vi "HE_state.vi"(6 "ZB":bool[](array[boolean])=[FALSE, FALSE], 7 "Alarm":bool[](array[boolean])=[FALSE, FALSE], 9 "XB":bool[](array[boolean])=[FALSE, FALSE, FALSE, FALSE, FALSE], 10 "Z_control":T5={"Z_HSw"=1, "Z_HSetState"=enum."on", "Z_ASetState"=enum."on", "Z_DSetState"=enum."on"}, 11 "HE_state_in":refnum<class "HE_state_v2.lvclass">) -> (1 "YB":bool[](array[boolean]), 2 "Z":T1={"Z_Source"=enum."local disabled", "Z_SetState"=enum."on", "Z_State"=enum."alarm", "Z_State_T"=0, "ZM_State"=enum."initialization", "ZM_State_T"=0, "ALR  L1"=FALSE, "ALR  L2"=FALSE, "HH_run"=0}, 3 "HE_state_out":refnum<class "HE_state_v2.lvclass">, 5 "ALR_ON":bool[](array[boolean]))   [LabVIEW 2019, in "Heating.lvlib" / "HE_state_v2.lvclass"]
uses:
  HE_state_v2.lvclass
  Heating.lvlib
  ctl/ZM_State.ctl
  ctl/Z_State.ctl
  ctl/Z_source.ctl
  ctl/Z.ctl
  ZM_state/HE_ZM_state.lvclass
  Z_state_v2/HE_Z_state_v2.lvclass
  C:/my_projects/projects/Algorithms/Labview/19/Heating/heating1/Z_state_v2/HE_Z_state_v2.lvclass
  C:/my_projects/projects/Algorithms/Labview/19/Heating/heating1/ZM_state/HE_ZM_state.lvclass
  C:/my_projects/projects/Algorithms/Labview/19/Sequence/State/State.lvclass
  ctl/Z_control.ctl
panel:
  # "Alarm_L1"
  # "Alarm_L2"
  # "Ki_XB01 contactor on"
  # "Ki_XB02 contactor off"
  # "XB24 local hand on"
  # "heating end"
  # "cooling end"
  # "Ki_ZB01 contactor on reg"
  # "Ki_ZB02 contactor off reg"
  # "TsStop"
  # "T_check"
  # "T_start_delay"
  # "T_heat_start"
  # "T_stop_delay"
  # "T_set_min"
  # "T_heat_stop"
  # "T_restart_delay"
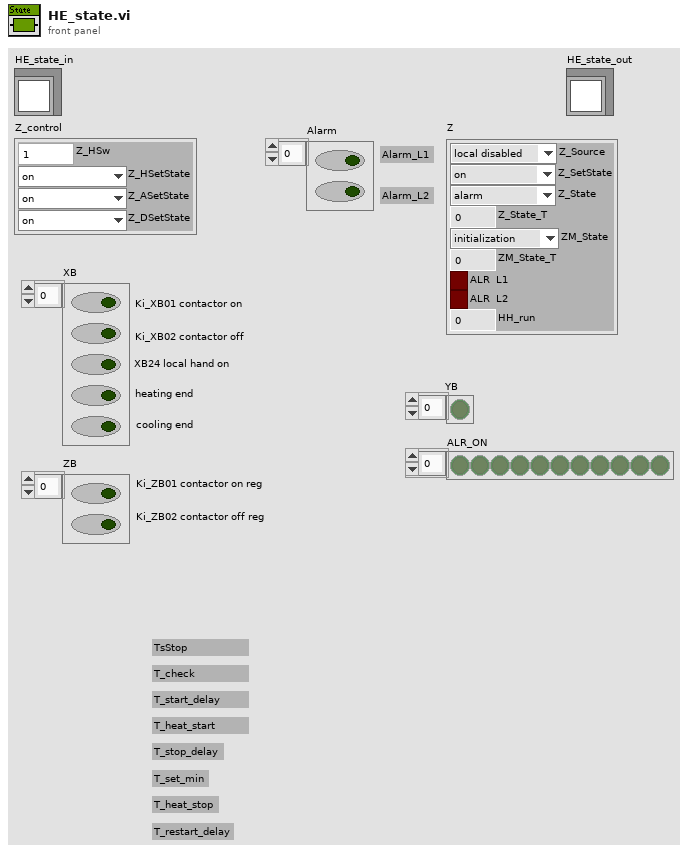
[diagram p1: front panel]
types:
  T1 = typedef "Heating.lvlib/Z.ctl" = cluster{"Z_Source":T2, "Z_SetState":T3, "Z_State":T3, "Z_State_T":u32, "ZM_State":T4, "ZM_State_T":u32, "ALR  L1":bool, "ALR  L2":bool, "HH_run":u64}
  T2 = typedef "Heating.lvlib/Z_source.ctl" = enum8{"initialize", "local disabled", "local hand", "hand", "auto", "dist"}
  T3 = typedef "Heating.lvlib/Z_State.ctl" = enum8{"initialization", "alarm", "disabled", "not ready", "stop ready", "reserv", "switched off", "reserv2", "switched on", "check", "on min", "decrease out", "on", "increase out", "on max"}
  T4 = typedef "Heating.lvlib/ZM_State.ctl" = enum8{"initialization", "stop", "start_cmd", "contactor_on_cmd", "heating", "on", "stop_cmd", "power_down", "contactor_off_cmd", "cooling", "restart_delay"}
  T5 = typedef "Heating.lvlib/Z_control.ctl" = cluster{"Z_HSw":u8, "Z_HSetState":T3, "Z_ASetState":T3, "Z_DSetState":T3}
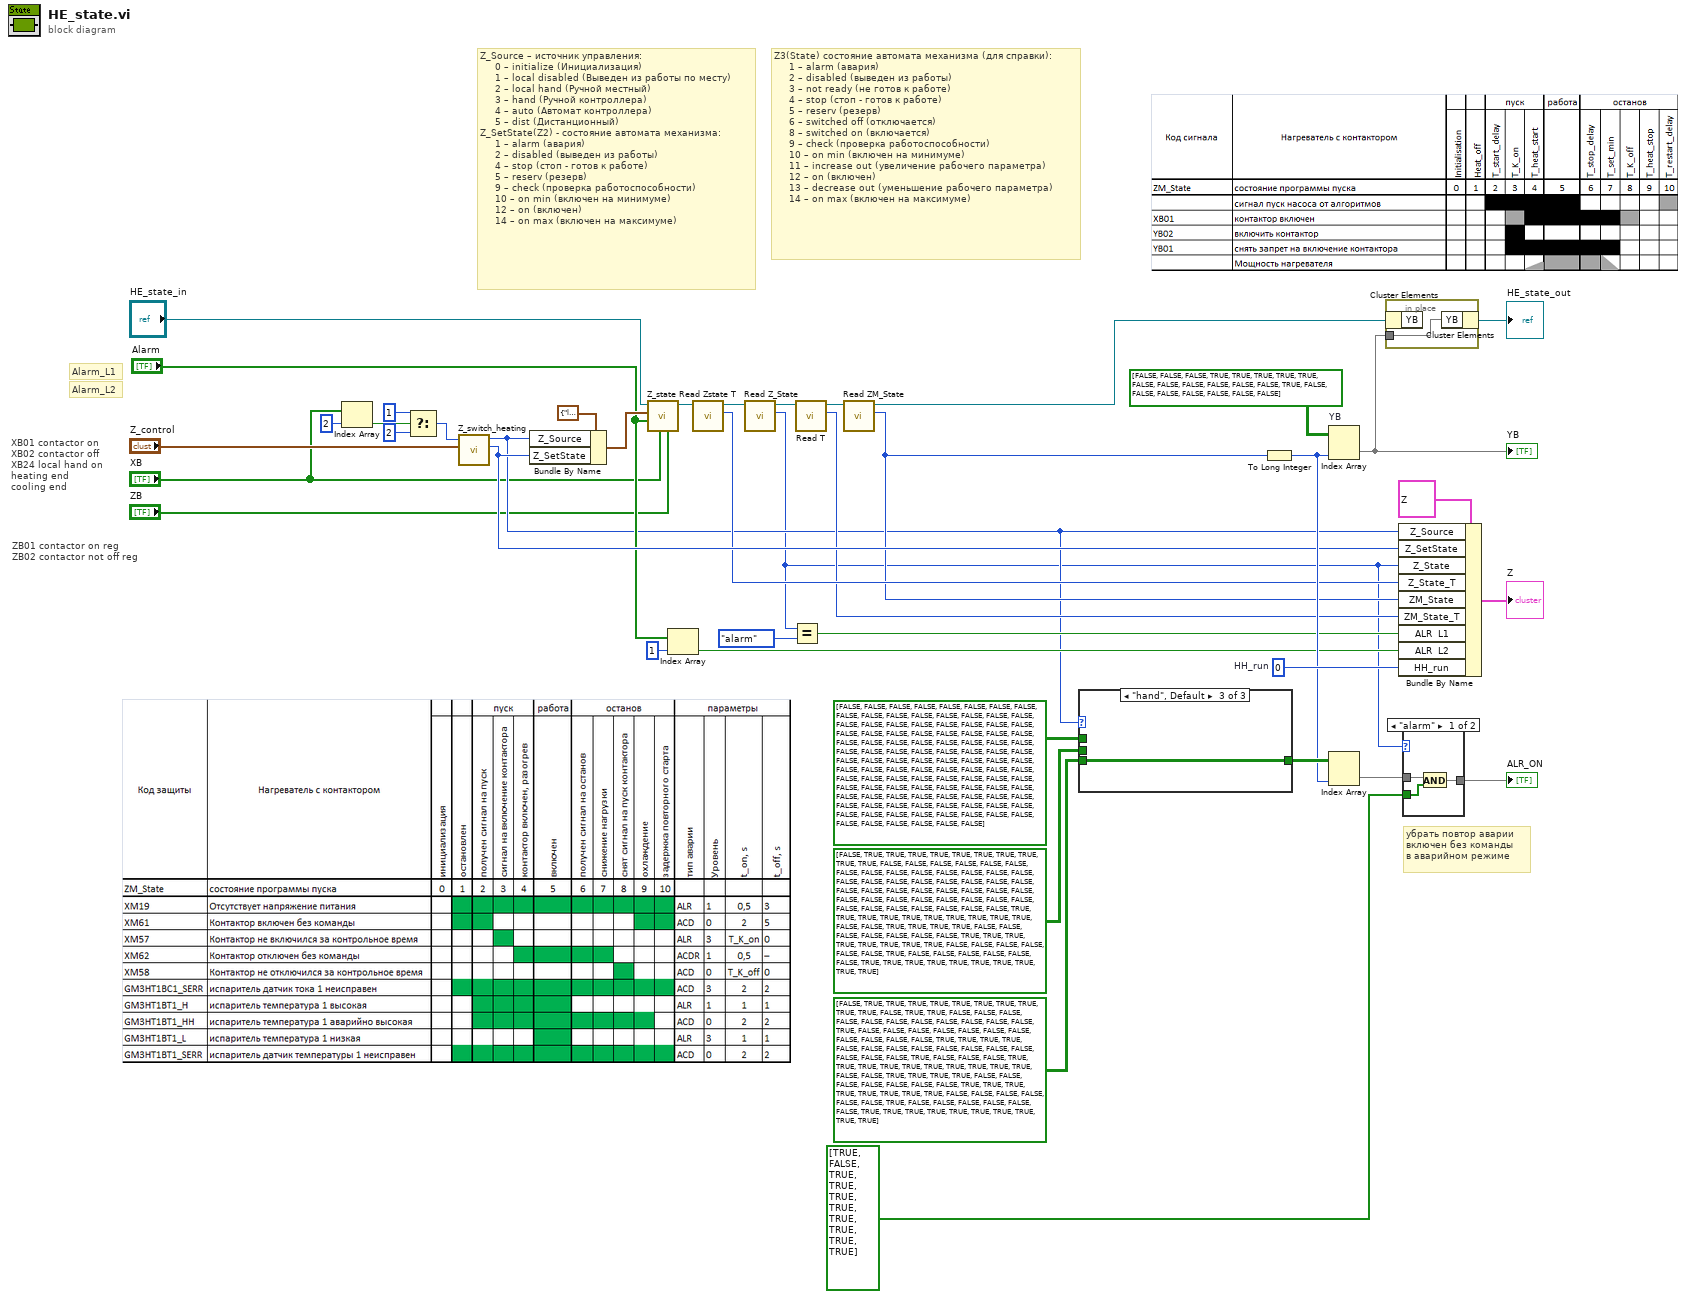
[diagram p0: block diagram]
diagram:
  w25 = 0  # HH_run
  # "Alarm_L2"
  # "Alarm_L1"
  # "ZB01 contactor on reg\nZB02 contactor not off reg"
  # "XB01 contactor on\nXB02 contactor off\nXB24 local hand on\nheating end\ncooling end"
  # "убрать повтор аварии\nвключен без команды\nв аварийном режиме"
  # "Z_Source – источник управления:\n     0 – initialize (Инициализация)\n     1 – local disabled (Выведен из работы по месту)\n     2 – local hand (Ручной местный)\n     3 – hand (Ручной контроллера)\n     4 – auto (Автомат контроллера)\n     5 – dist (Дистанционный)\nZ_SetState(Z2) - состояние автомата механизма:\n     1 – alarm (авария)\n     2 – disabled (выведен из работы)\n     4 – stop (стоп - готов к работе)\n     5 – reserv (резерв)\n     9 – check (проверка работоспособности)\n     10 – on min (включен на минимуме)\n     12 – on (включен)\n     14 – on max (включен на максимуме)"
  # "Z3(State) состояние автомата механизма (для справки):\n     1 – alarm (авария)\n     2 – disabled (выведен из работы)\n     3 – not ready (не готов к работе)\n     4 – stop (стоп - готов к работе)\n     5 – reserv (резерв)\n     6 – switched off (отключается)\n     8 – switched on (включается)\n     9 – check (проверка работоспособности)\n     10 – on min (включен на минимуме)\n     11 – increase out (увеличение рабочего параметра)\n     12 – on (включен)\n     13 – decrease out (уменьшение рабочего параметра)\n     14 – on max (включен на максимуме)"
  n1 = Index Array(array="XB", index=2) -> (element=w27:bool)
  n2 = Select(t=u8 1, s=w27, f=u8 2) -> (s? t:f=w35:u8)
  n3 = call "Z_switch_heating.vi"("Z"="Z_control", "Z_LSw"=w35) -> ("Z_SetState"=w18:T3, "Z_Source"=w10:T2)  [unwired: 8 in]
  n4 = Bundle By Name(cluster=cluster{"Z_Source":T2, "Z_SetState":T3} {"Z_Source"=enum."local disabled", "Z_SetState"=enum."alarm"} ("Z_In"), "Z_Source"=w10, "Z_SetState"=w18) -> (w17:cluster{"Z_Source":T2, "Z_SetState":T3})
  n5 = call "Z_state.vi"("ZB"="ZB", "XB"="XB", "Alarm"="Alarm", "Z_In"=w17, "HE1_Z_state in"="HE_state_in") -> ("HE1_Z_state out"=w3:refnum<class "HE_state_v2.lvclass">)  [unwired: 6 in]
  n6 = Index Array(array="Alarm", index=1) -> (element=w20:bool)
  n7 = call "Read Zstate T.vi"("HE1_Z_state in"=w3) -> ("T (ms)"=w14:u32, "HE1_Z_state out"=w15:refnum<class "HE_state_v2.lvclass">)  [unwired: 9 in]
  n8 = call "Read Z_State.vi"("HE1_Z_state in"=w15) -> ("Z_State_heating"=w4:T3, "HE1_Z_state out"=w2:refnum<class "HE_state_v2.lvclass">)  [unwired: 9 in]
  n9 = Equal?(x=w4, y=Z_State."alarm") -> (x = y?=w22:bool)
  n10 = call "Read T.vi"("valve_VCH_ZM_state in"=w2) -> ("T (ms)"=w11:u32, "valve_VCH_ZM_state out"=w13:refnum<class "HE_state_v2.lvclass">)  [unwired: 9 in]
  n11 = call "Read ZM_State.vi"("HE_ZM_state in"=w13) -> ("ZM_State"=w12:T4, "HE_ZM_state out"=w1:refnum<class "HE_state_v2.lvclass">)  [unwired: 9 in]
  n12 = case shown="\"hand\", Default" w10 {
    tunnel: bool[][] [[FALSE, FALSE, FALSE, FALSE, FALSE, FALSE, FALSE, FALSE, FALSE, FALSE, FALSE], [FALSE, FALSE, FALSE, FALSE, FALSE, FALSE, FALSE, FALSE, FALSE, FALSE, FALSE], [FALSE, FALSE, FALSE, FALSE, FALSE, FALSE, FALSE, FALSE, FALSE, FALSE, FALSE], [FALSE, FALSE, FALSE, FALSE, FALSE, FALSE, FALSE, FALSE, FALSE, FALSE, FALSE], [FALSE, FALSE, FALSE, FALSE, FALSE, FALSE, FALSE, FALSE, FALSE, FALSE, FALSE], [FALSE, FALSE, FALSE, FALSE, FALSE, FALSE, FALSE, FALSE, FALSE, FALSE, FALSE], [FALSE, FALSE, FALSE, FALSE, FALSE, FALSE, FALSE, FALSE, FALSE, FALSE, FALSE], [FALSE, FALSE, FALSE, FALSE, FALSE, FALSE, FALSE, FALSE, FALSE, FALSE, FALSE], [FALSE, FALSE, FALSE, FALSE, FALSE, FALSE, FALSE, FALSE, FALSE, FALSE, FALSE], [FALSE, FALSE, FALSE, FALSE, FALSE, FALSE, FALSE, FALSE, FALSE, FALSE, FALSE]] -> [w42 _ _]
    tunnel: bool[][] [[FALSE, TRUE, TRUE, TRUE, TRUE, TRUE, TRUE, TRUE, TRUE, TRUE, TRUE], [FALSE, FALSE, FALSE, FALSE, FALSE, FALSE, FALSE, FALSE, FALSE, FALSE, FALSE], [FALSE, FALSE, FALSE, FALSE, FALSE, FALSE, FALSE, FALSE, FALSE, FALSE, FALSE], [FALSE, FALSE, FALSE, FALSE, FALSE, FALSE, FALSE, FALSE, FALSE, FALSE, FALSE], [FALSE, FALSE, FALSE, FALSE, FALSE, FALSE, FALSE, FALSE, FALSE, FALSE, FALSE], [FALSE, TRUE, TRUE, TRUE, TRUE, TRUE, TRUE, TRUE, TRUE, TRUE, TRUE], [FALSE, FALSE, TRUE, TRUE, TRUE, TRUE, FALSE, FALSE, FALSE, FALSE, FALSE], [FALSE, FALSE, TRUE, TRUE, TRUE, TRUE, TRUE, TRUE, TRUE, TRUE, FALSE], [FALSE, FALSE, FALSE, FALSE, FALSE, TRUE, FALSE, FALSE, FALSE, FALSE, FALSE], [FALSE, TRUE, TRUE, TRUE, TRUE, TRUE, TRUE, TRUE, TRUE, TRUE, TRUE]] -> [_ w43 _]
    tunnel: bool[][] [[FALSE, TRUE, TRUE, TRUE, TRUE, TRUE, TRUE, TRUE, TRUE, TRUE, TRUE], [FALSE, TRUE, TRUE, FALSE, FALSE, FALSE, FALSE, FALSE, FALSE, FALSE, FALSE], [FALSE, FALSE, FALSE, TRUE, FALSE, FALSE, FALSE, FALSE, FALSE, FALSE, FALSE], [FALSE, FALSE, FALSE, FALSE, TRUE, TRUE, TRUE, TRUE, FALSE, FALSE, FALSE], [FALSE, FALSE, FALSE, FALSE, FALSE, FALSE, FALSE, FALSE, TRUE, FALSE, FALSE], [FALSE, TRUE, TRUE, TRUE, TRUE, TRUE, TRUE, TRUE, TRUE, TRUE, TRUE], [FALSE, FALSE, TRUE, TRUE, TRUE, TRUE, FALSE, FALSE, FALSE, FALSE, FALSE], [FALSE, FALSE, TRUE, TRUE, TRUE, TRUE, TRUE, TRUE, TRUE, TRUE, FALSE], [FALSE, FALSE, FALSE, FALSE, FALSE, TRUE, FALSE, FALSE, FALSE, FALSE, FALSE], [FALSE, TRUE, TRUE, TRUE, TRUE, TRUE, TRUE, TRUE, TRUE, TRUE, TRUE]] -> [_ _ w44]
    tunnel: [w42 w43 w44] -> w39
    frame "initialize", "local disabled" {
    }
    frame "local hand" {
    }
    frame "hand", Default {
    }
  }
  n13 = To Long Integer(number=w12) -> (32bit integer=w24:i32)
  n14 = Index Array "YB"(array=bool[][] [[FALSE, FALSE, FALSE, TRUE, TRUE, TRUE, TRUE, TRUE, FALSE, FALSE, FALSE], [FALSE, FALSE, FALSE, TRUE, FALSE, FALSE, FALSE, FALSE, FALSE, FALSE, FALSE]], index (col)=w24) -> (element=w9:bool[])  [unwired: 1 in]
  "YB" <- w9
  n15 = Index Array(array=w39, index (col)=w24) -> (element=w38:bool[])  [unwired: 1 in]
  n16 = in-place {
    in-place-border: w9 -> [w45]
    n17 = in-place-cluster #1(w1) -> ()  [unwired: 1 out]
    n18 = in-place-cluster #1("YB"=w45) -> (→"HE_state_out":refnum<class "HE_state_v2.lvclass">)
  }
  n19 = Bundle By Name(cluster=T1 {"Z_Source"=enum."local disabled", "Z_SetState"=enum."on", "Z_State"=enum."alarm", "Z_State_T"=0, "ZM_State"=enum."initialization", "ZM_State_T"=0, "ALR  L1"=FALSE, "ALR  L2"=FALSE, "HH_run"=0} ("Z"), "Z_Source"=w10, "Z_SetState"=w18, "Z_State"=w4, "Z_State_T"=w14, "ZM_State"=w12, "ZM_State_T"=w11, "ALR  L1"=w22, "ALR  L2"=w20, "HH_run"=w25) -> (→"Z":T1)
  n20 = case shown="\"alarm\"" w4 {
    tunnel: bool[] [TRUE, FALSE, TRUE, TRUE, TRUE, TRUE, TRUE, TRUE, TRUE, TRUE] -> [w47 _]
    tunnel: w38 -> [w48 w49]
    tunnel: [w46 w49] -> w37
    frame "alarm" {
      n21 = And(x=w48, y=w47) -> (x .and. y?=w46:bool[])
    }
    frame "disabled", Default {
    }
  }
  "ALR_ON" <- w37
